vi "Connect Set-PVs.vi"(8 "Error In":errorcluster, 10 "Set-Messages":T1(array[cluster]), 11 "CS++GUIActor in":refnum<class "CS++GUIActor.lvclass">) -> (0 "Error Out":errorcluster, 2 "PVConnections":refnum<class "PVConnection.lvclass">[](array[class]), 3 "CS++GUIActor out":refnum<class "CS++GUIActor.lvclass">)   [LabVIEW 2015, in "CS++GUIActor.lvlib" / "CS++GUIActor.lvclass"]
doc: "Opens the connection to (already existing) PVs to set values."
uses:
  CS++GUIActor.lvclass
  Classes/CS++ProcessVariables/PVConnection/PVConnection.lvclass
  CS++BaseActor/CS++BaseActor.lvclass/CS++BaseActor.ctl
  CS++GUIActor.lvclass/CS++GUIActor.ctl
  Classes/CS++ProcessVariables/ProcessVariable/PV.lvclass
  Classes/CS++ProcessVariables/PV Type.ctl
  Classes/CS++ProcessVariables/ProcessVariable/PV.lvclass/PV.ctl
  Classes/CS++ProcessVariables/ProcessVariable/Write Name.vi
  Classes/CS++ProcessVariables/ProcessVariable/Write PV URL.vi
  Classes/CS++ProcessVariables/ProcessVariable/Write Type Descriptor.vi
  Classes/CS++ProcessVariables/ProcessVariable/Write PV Type.vi
  CS++BaseActor/Read CS++Factory.vi
  Read Associated Proxy Actor Name.vi
  <vilib>/Utility/error.llb/Error Cluster From Error Code.vi
  Classes/CS++BaseClasses/Factory/CS++Factory.lvclass
  Classes/CS++ProcessVariables/CS++ProcessVariables.lvlib
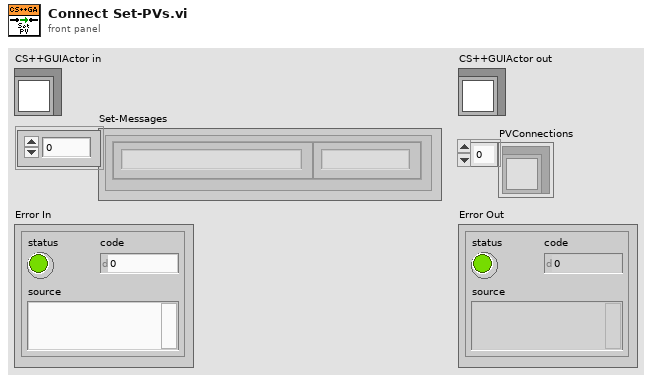
[diagram p1: front panel]
types:
  T1 = cluster{"Message Name":string, "Datatype Desciptor":string}[]
  T2 = typedef "CS++ProcessVariables.lvlib/PV Type.ctl" = enum16{"Service", "Command"}
  T3 = cluster{"Read Access":enum8{"Allowed", "Required", "None"}, "Write Access":enum8{"Allowed", "Required", "None"}}
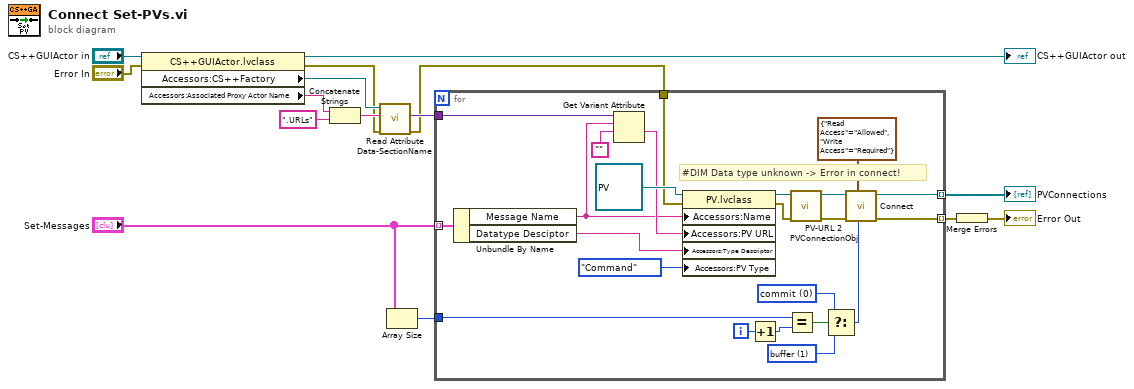
[diagram p0: block diagram]
diagram:
  n1 = property class="CS++GUIActor.lvclass"(reference="CS++GUIActor in", error in="Error In") -> (reference out=→"CS++GUIActor out":refnum<class "CS++GUIActor.lvclass">, error out=w4:errorcluster, "Accessors:CS++Factory"=w8:refnum<class "CS++Factory.lvclass">, "Accessors:Associated Proxy Actor Name"=w10:string)
  n2 = Concatenate Strings(w10, ".URLs" ("Object Name")) -> (w9:string)
  n3 = call-dynamic "Read Attribute Data-SectionName.vi"("error in (no error)"=w4, "Object Name"=w9, "CS++Factory in"=w8) -> ("error out"=w3:errorcluster, "Attribute Data"=w12:variant)  [unwired: 6 in, 1 out]
  n4 = Array Size(array="Set-Messages") -> (size(s)=w1:i32)
  n5 = for {
    tunnel: w3 -> [w32]
    tunnel: w12 -> [w31]
    tunnel: "Set-Messages" -> [w18] mode=indexing
    tunnel: w1 -> [w27]
    tunnel: [w21] -> w7 mode=indexing
    tunnel: [w20] -> w6 mode=indexing
    i -> [w28]
    w24 = u16 0 items=["commit", "buffer"] ("Mode (buffer)")
    w23 = u16 1 items=["commit", "buffer"] ("Mode (buffer)")
    # "#DIM Data type unknown -> Error in connect!"
    n6 = Unbundle By Name(w18) -> ("Message Name"=w17:string, "Datatype Desciptor"=w16:string)
    n7 = Get Variant Attribute(Variant=w31, name=w17, default value (empty Variant)="") -> (value=w29:string)  [unwired: 1 in, 3 out]
    n8 = property class="PV.lvclass"(reference=refnum<class "PV.lvclass"> refnum ("CS++ProcessVariables.lvlib:PV.lvclass"), error in=w32, "Accessors:Name"=w17, "Accessors:PV URL"=w29, "Accessors:Type Descriptor"=w16, "Accessors:PV Type"=PV_Type."Command" ("PV Type")) -> (reference out=w36:refnum<class "PV.lvclass">, error out=w34:errorcluster)
    n9 = Increment(x=w28) -> (x+1=w26:i32)
    n10 = Equal?(x=w27, y=w26) -> (x = y?=w25:bool)
    n11 = call "PV-URL 2 PVConnectionObj.vi"("Error In"=w34, "PV"=w36) -> ("Error Out"=w38:errorcluster, "PVConnection"=w37:refnum<class "PVConnection.lvclass">)  [unwired: 7 in, 1 out]
    n12 = Select(t=w24, s=w25, f=w23) -> (s? t:f=w22:u16)
    n13 = call "Connect.vi"("Access (R/W allowed)"=T3 {"Read Access"=enum."Allowed", "Write Access"=enum."Required"}, "Mode (buffer)"=w22, "Error In"=w38, "PVConnection in"=w37) -> ("Error Out"=w20:errorcluster, "PVConnection out"=w21:refnum<class "PVConnection.lvclass">)  [unwired: 6 in]
  }
  "PVConnections" <- w7
  n14 = Merge Errors(w6) -> (→"Error Out":errorcluster)
